vi "PXI-Ramp Bank.vi"(0 "Action":enum16{"Add", "Read", "Clear"}(ring), 7 "Ramp In":dbl[](array[numeric]) format="%.2f") -> (4 "Ramp available?":bool, 8 "Ramp Out":dbl[](array[numeric]) format="%.2f")   [LabVIEW 2020]
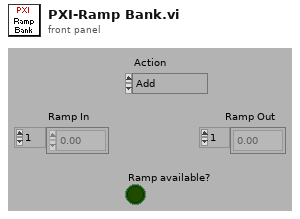
[diagram p1: front panel]
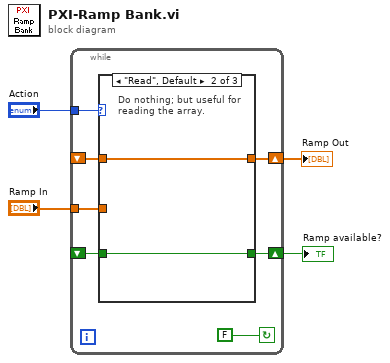
[diagram p0: block diagram]
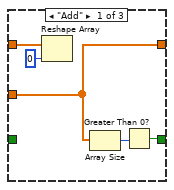
[diagram p2: hidden frame]
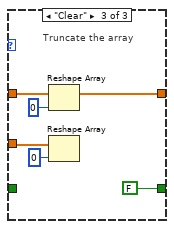
[diagram p3: hidden frame]
diagram:
  n1 = while {
    tunnel: "Ramp In" -> [w7]
    shift-left: _ -> [w9]
    shift-right: [w8] -> w2
    shift-left: _ -> [w6]
    shift-right: [w10] -> w1
    tunnel: "Action" -> [w11]
    stop <- FALSE continue-if-true
    n2 = case shown="\"Read\", Default" w11 {
      tunnel: w6 -> [w15 w17 w24]
      tunnel: [w14 w17 w19] -> w10
      tunnel: w9 -> [_ w18 _]
      tunnel: [w12 w18 FALSE] -> w8
      tunnel: w7 -> [w14 _ w21]
      frame "Add" {
        n3 = Reshape Array(w15, 0) -> ()  [unwired: 1 out]
        n4 = Array Size(array=w14) -> (size(s)=w13:i32)
        n5 = Greater Than 0?(x=w13) -> (x > 0?=w12:bool)
      }
      frame "Read", Default {
        # "Do nothing; but useful for\nreading the array."
      }
      frame "Clear" {
        # "Truncate the array"
        n6 = Reshape Array(w24, 0) -> (w19:dbl[])
        n7 = Reshape Array(w21, 0 ("dimension size")) -> ()  [unwired: 1 out]
      }
    }
  }
  "Ramp Out" <- w1
  "Ramp available?" <- w2
